vi "Configure Measurement Delay.vi"(6 "Delay Factor (0 S)":dbl, 7 "Delay Type (0: Measurement Delay)":i32(ring) items=["Measurement Delay", "High Capacitance Mode Delay"], 8 "error in (no error)":errorcluster, 9 "Delay Time (0 S)":dbl, 10 "Source Measure Unit Channel (0: Channel A)":i32(ring) items=["Channel A", "Channel B"], 11 "VISA resource name":refnum<visa-resource-name>) -> (0 "error out":errorcluster, 3 "VISA resource name out":refnum<visa-resource-name>)   [LabVIEW 2020, in "Keithley 2600 Series.lvlib"]
doc: "Configures the measurement delay time."
uses:
  <instrlib>/Keithley 2600 Series/Keithley 2600 Series.lvlib
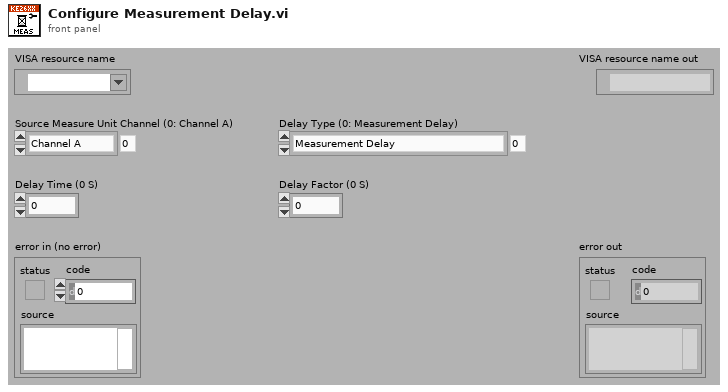
[diagram p1: front panel]
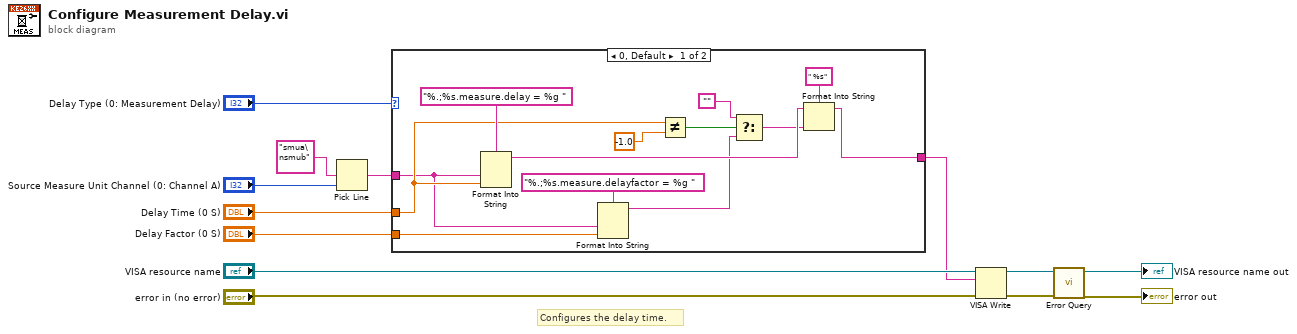
[diagram p0: block diagram]
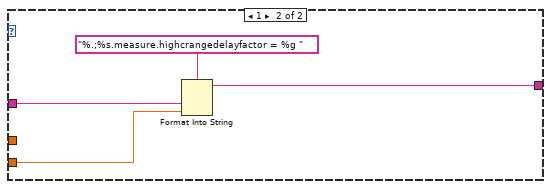
[diagram p2: hidden frame]
diagram:
  # "Configures the delay time."
  n1 = Pick Line(multi-line string="smua\nsmub", line index="Source Measure Unit Channel (0: Channel A)") -> (output string=w4:string)  [unwired: 1 in]
  n2 = case shown="0, Default" "Delay Type (0: Measurement Delay)" {
    tunnel: "Delay Time (0 S)" -> [w25 _]
    tunnel: w4 -> [w22 w29]
    tunnel: "Delay Factor (0 S)" -> [w23 w28]
    tunnel: [w14 w27] -> w1
    frame 0, Default {
      n3 = Format Into String(format string="%.;%s.measure.delay = %g ", w22, w25) -> (resulting string=w19:string)  [unwired: 2 in, 1 out]
      n4 = Format Into String(format string="%.;%s.measure.delayfactor = %g ", w22, w23) -> (resulting string=w17:string)  [unwired: 2 in, 1 out]
      n5 = Not Equal?(x=w25, y=-1.0) -> (x != y?=w20:bool)
      n6 = Select(t="", s=w20, f=w17) -> (s? t:f=w16:string)
      n7 = Format Into String(format string=" %s", initial string=w19, w16) -> (resulting string=w14:string)  [unwired: 1 in, 1 out]
    }
    frame 1 {
      n8 = Format Into String(format string="%.;%s.measure.highcrangedelayfactor = %g ", w29, w28) -> (resulting string=w27:string)  [unwired: 2 in, 1 out]
    }
  }
  n9 = VISA Write(VISA resource name="VISA resource name", write buffer=w1, error in (no error)="error in (no error)") -> (VISA resource name out=w11:refnum<visa-resource-name>, error out=w10:errorcluster)  [unwired: 1 out]
  n10 = call <instrlib>:"Error Query.vi"("error in (no error)"=w10, "VISA resource name"=w11) -> ("error out"=→"error out":errorcluster, "VISA resource name out"=→"VISA resource name out":refnum<visa-resource-name>)  [unwired: 6 in, 2 out]
